vi "solve_quadratic_equation.vi"(8 "error in (no error)":errorcluster, 9 "c":dbl, 10 "b":dbl, 11 "a":dbl) -> (0 "error out":errorcluster, 2 "x2 (smaller result)":dbl, 3 "x1 (bigger result)":dbl)   [LabVIEW 2010]
uses:
  <vilib>/express/express arith-compare/Formula/XNode/ExpressFormulaBlockNode.xnode
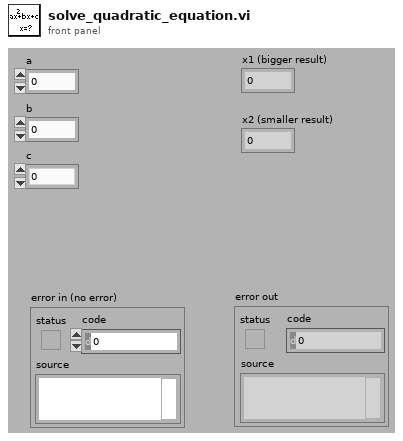
[diagram p1: front panel]
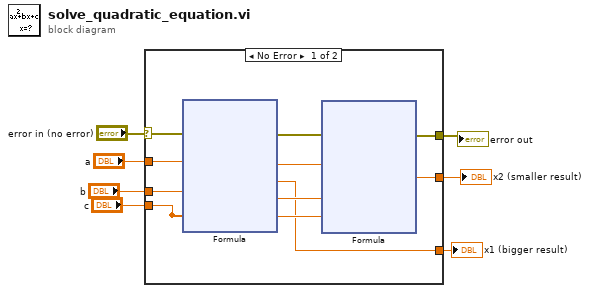
[diagram p0: block diagram]
diagram:
  n1 = case shown="No Error" "error in (no error)" {
    selector: "error in (no error)" -> [w15 w40]
    tunnel: "b" -> [w11 _]
    tunnel: "a" -> [w12 _]
    tunnel: "c" -> [w10 _]
    tunnel: [w13 w40] -> w3
    tunnel: [w9 _] -> w2
    tunnel: [w8 _] -> w1
    frame No Error {
      n2 = xnode "Formula"("a"=w12, "b"=w11, "c"=w10, "error in (no error)"=w15) -> ("Result"=w9:dbl, "error out"=w14:errorcluster)
      n3 = xnode "Formula"("a"=w12, "b"=w11, "c"=w10, "error in (no error)"=w14) -> ("Result"=w8:dbl, "error out"=w13:errorcluster)
    }
    frame Error {
    }
  }
  "error out" <- w3
  "x1 (bigger result)" <- w2
  "x2 (smaller result)" <- w1
